vi "Qudi_HiM_QPD_PID.vi"(3 "N Z positions":i32) -> ()   [LabVIEW 2015]
uses:
  <vilib>/rvi/Analysis/control/PID/Typedef/niFpgaPID_PIGains.ctl
  <vilib>/Platform/TimedLoop/XDataNode/timing_clust.ctl
  <vilib>/Platform/TimedLoop/XDataNode/nitl_modes.ctl
  <vilib>/Platform/TimedLoop/XDataNode/wakeup.ctl
  <vilib>/rvi/FXPMathLib/basic elements/FxpIntAccumulator/subVIs/nifxpmath_IntAccumulator_SimConfig.ctl
  <vilib>/rvi/Emulation/niFpgaGetClockAttributes.vi
  <vilib>/rvi/Emulation/niFpgaSctlEmulationGetInTimedLoop.vi
  <vilib>/rvi/Emulation/niFpgaEmulationReportErrorSimple.vi
  <vilib>/rvi/eio/common/nirviEmuTemplateMethod_errors.vi
  <vilib>/rvi/Emulation/niFpgaProcessEmulError.vi
  <vilib>/rvi/Analysis/common/codeGenErrors/XNode/niFpgaXNodeCodeGenErrorHandle.vi
  <vilib>/rvi/Emulation/niFpgaCriticalErrorInLSC.vi
  <vilib>/rvi/FXPMathLib/basic elements/FxpIntAccumulator/simVIs/DllFxpIntAccumulator_sub.vi
  <vilib>/rvi/Analysis/control/PID/SubVIs/niFpgaPID_PIWrapper.vi
  <vilib>/eio/EIONode/EIONode.xnode
  <vilib>/rvi/Analysis/measure/dc-rms/XNode/niFpgaDC-RMS.xnode
  <vilib>/Platform/TimedLoop/XDataNode/XDataNode.xnode
  <vilib>/rvi/FXPMathLib/basic elements/FxpIntAccumulator/XNode/nifxpmath_IntAccumulator.xnode
  <vilib>/Platform/TimedLoop/XDataNode/XDNodeRunTimeDep.lvlib
panel:
  in  "exposure_time_ms":u16
  in  "integration_time_us":u32=100 caption="Count(uSec)"
  in  "stop":bool
  out "duration_ms":u32
  out "X":i16
  out "Y":i16
  out "Sum":i16
  out "counter":u32
  out "output":i16
  in  "reset":bool
  in  "reset_counter":bool
  in  "autofocus":bool
  in  "setpoint":i16
  in  "P":i16
  in  "I":i16
  in  "ref_axis":bool
  out "n cycles":i32
  out "Images acquired":i32
  in  "Laser lines":i32[](array[numeric])=[0, 0, 0, 0, 0]
  in  "Laser power":i16[](array[numeric])=[0, 0, 0, 0, 0]
  in  "N laser lines":i32
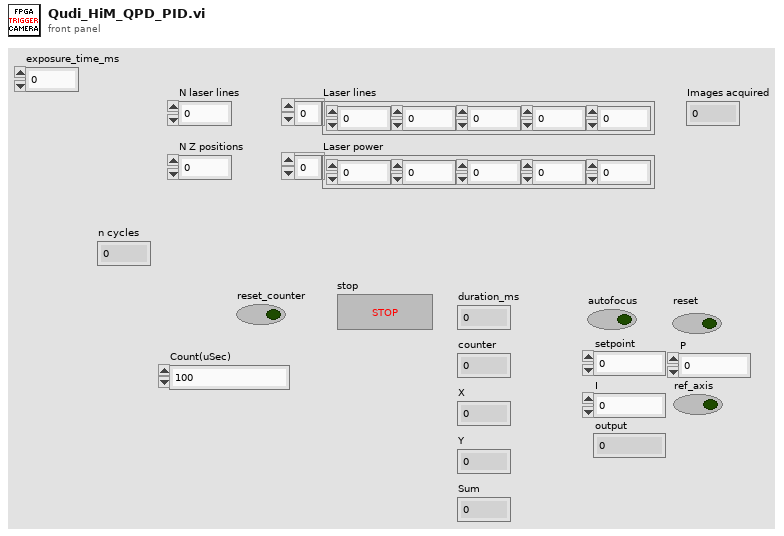
[diagram p1: front panel]
types:
  T1 = typedef "niFpgaPID_PIGains.ctl" = cluster{"proportional gain":sgl, "integral gain":sgl}
  T2 = typedef "XDNodeRunTimeDep.lvlib/timing_clust.ctl" = cluster{"Expected End [f-1]":u64, "Actual End [f-1]":u64, "Finished Late? [f-1]":bool, "Expected End [i-1]":u64, "Actual End [i-1]":u64, "Finished Late? [i-1]":bool, "Expected Start [i]":u64, "Actual Start [i]":u64, "Expected Start [f]":u64, "Actual Start [f]":u64, "Source Name":string, "Structure Name":string, "Period":i64, "Deadline":i64, "Offset":i64, "Start":i64, "Priority":i32, "Timeout":i32, "Mode":T3, "Wakeup Reason":T4, "Error":errorcluster, "Source Type":string, "Secondary Source Type":string, "Global End Time":u64, "Global Start Time":u64, "Frame Duration":u64, "Iteration Duration":u64, "Assigned CPU":i32, "I/O Scan Engine Mode":u32}
  T3 = typedef "XDNodeRunTimeDep.lvlib/nitl_modes.ctl" = enum32{"No Change", "Process missed periods, maintain original phase", "Discard missed periods, maintain original phase", "Process missed periods, ignore original phase", "Discard missed periods, ignore original phase"}
  T4 = typedef "XDNodeRunTimeDep.lvlib/wakeup.ctl" = enum32{"Normal", "Aborted", "Asynchronous wakeup", "Timing source error", "Timed loop error", "Timeout"}
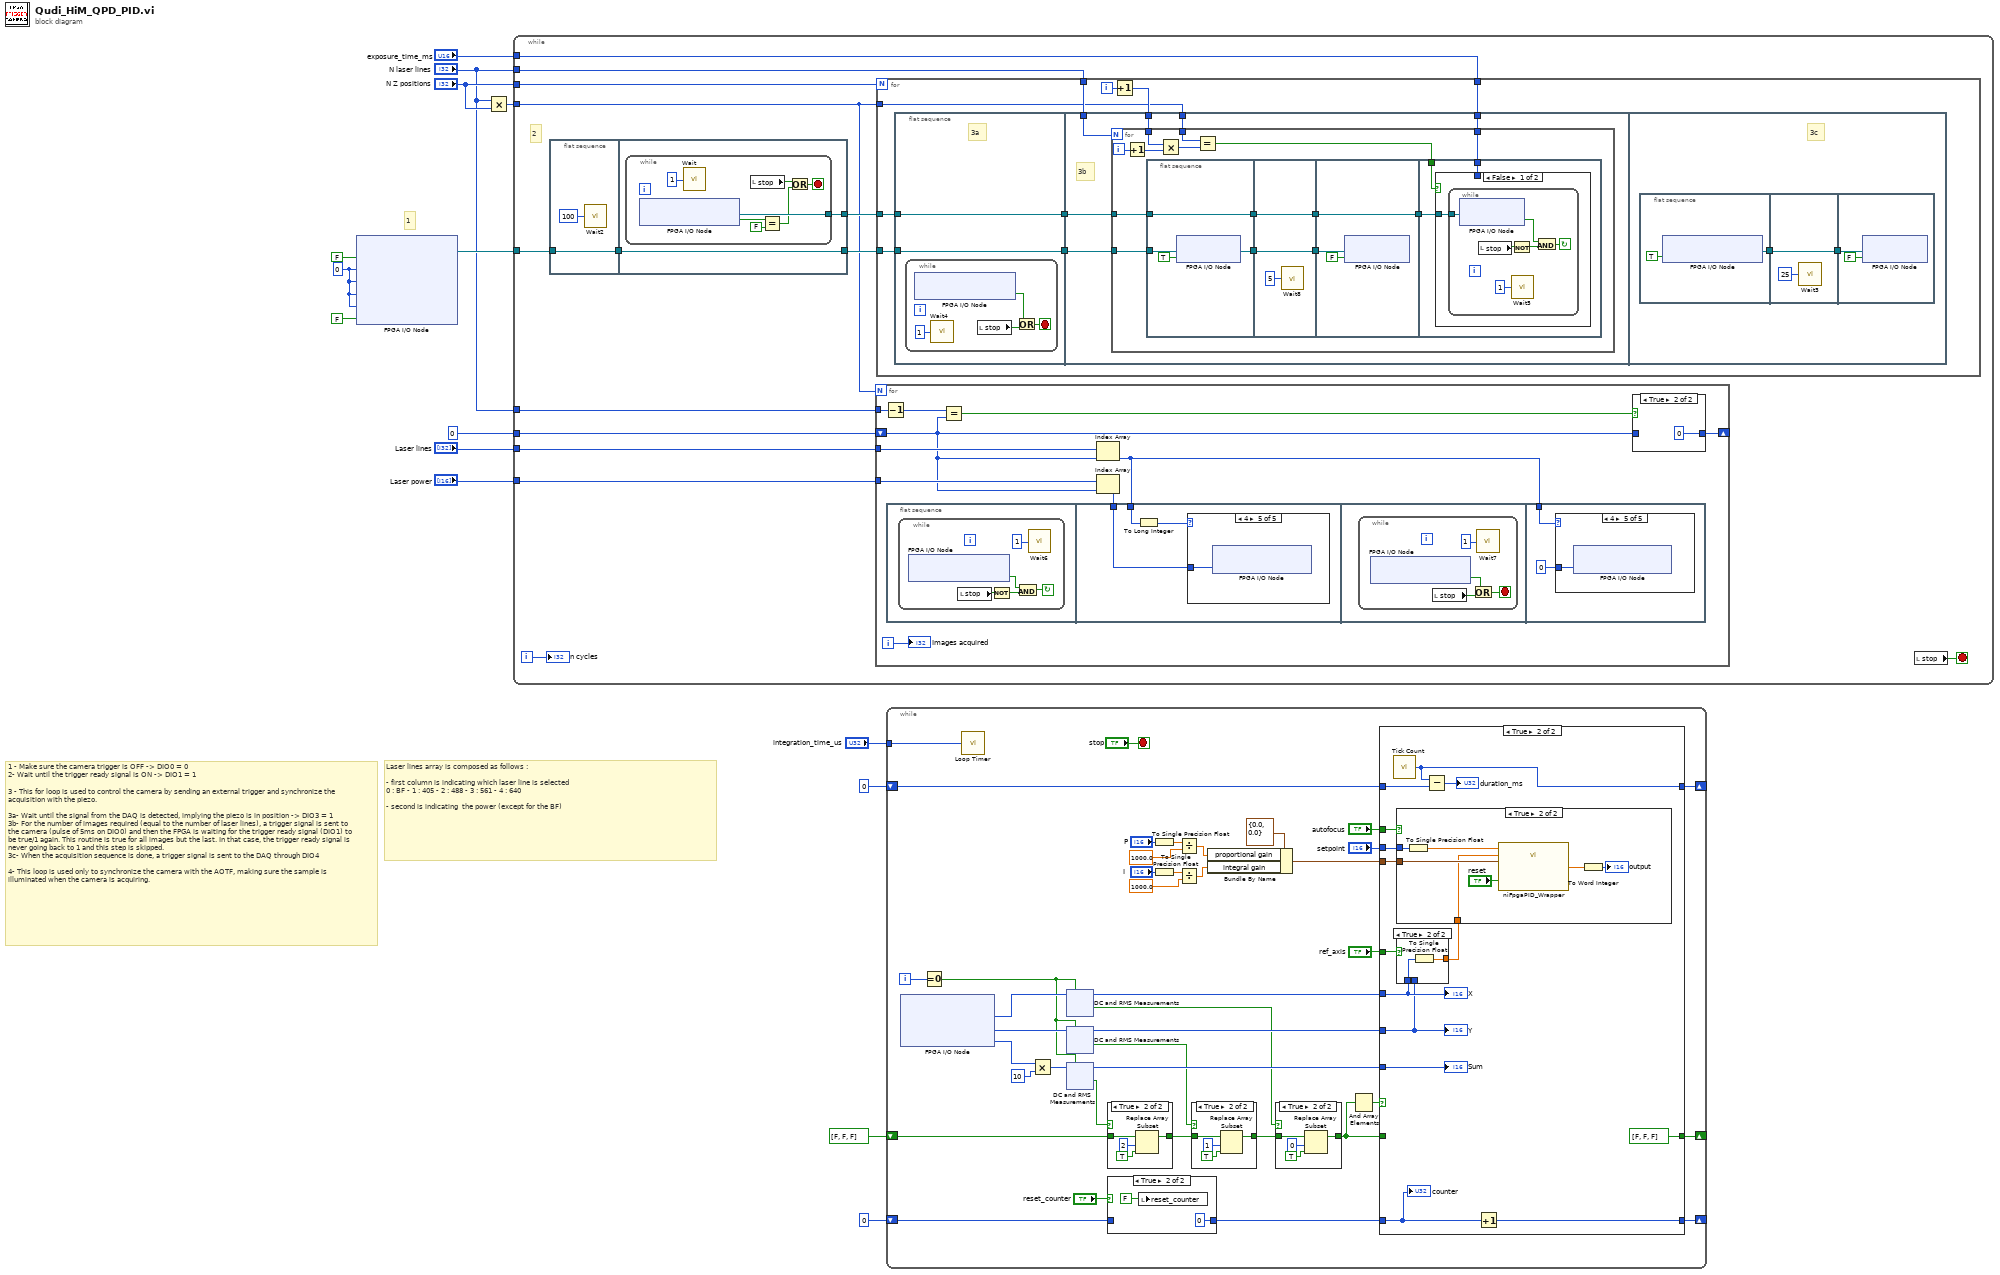
[diagram p0: block diagram]
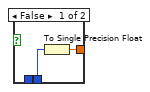
[diagram p7: hidden frame]
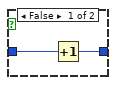
[diagram p9: hidden frame]
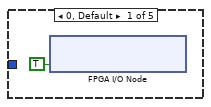
[diagram p10: hidden frame]
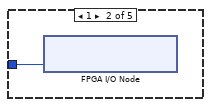
[diagram p11: hidden frame]
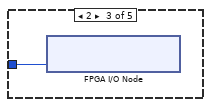
[diagram p12: hidden frame]
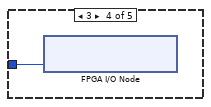
[diagram p13: hidden frame]
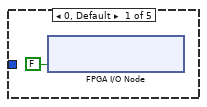
[diagram p14: hidden frame]
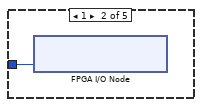
[diagram p15: hidden frame]
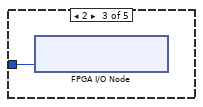
[diagram p16: hidden frame]
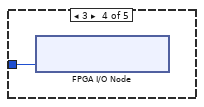
[diagram p17: hidden frame]
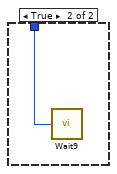
[diagram p18: hidden frame]
diagram:
  w10 = i16 0 ("Connector0/AO0")
  # "Laser lines array is composed as follows :\n\n- first column is indicating which laser line is selected \n0 : BF - 1 : 405 - 2 : 488 - 3 : 561 - 4 : 640\n\n- second is indicating  the power (except for the BF)"
  # "1"
  # "1 - Make sure the camera trigger is OFF -> DIO0 = 0\n2- Wait until the trigger ready signal is ON -> DIO1 = 1\n\n3 - This for loop is used to control the camera by sending an external trigger and synchronize the acquisition with the piezo.\n\n3a- Wait until the signal from the DAQ is detected, implying the piezo is in position -> DIO3 = 1 \n3b- For the number of images required (equal to the number of laser lines), a trigger signal is sent to the camera (pulse of 5ms on DIO0) and then the FPGA is waiting for the trigger ready signal (DIO1) to be true/1 again. This routine is true for all images but the last. In that case, the trigger ready signal is never going back to 1 and this step is skipped. \n3c- When the acquisition sequence is done, a trigger signal is sent to the DAQ through DIO4\n\n4- This loop is used only to synchronize the camera with the AOTF, making sure the sample is illuminated when the camera is acquiring."
  n1 = xnode "FPGA I/O Node"("Connector0/DIO0"=FALSE, "Connector0/AO0"=w10, "Connector0/AO1"=w10, "Connector0/AO2"=w10, "Connector0/AO3"=w10, "Connector0/DIO5"=FALSE) -> ("FPGA I/O Out"=w14:refnum<k21>)  [unwired: 6 in, 5 out]
  n2 = Multiply(x="N laser lines", y="N Z positions") -> (x*y=w3:i32)
  n3 = while {
    tunnel: w14 -> [w28]
    tunnel: "Laser power" -> [w25]
    tunnel: "Laser lines" -> [w24]
    tunnel: 0 -> [w23]
    tunnel: "N Z positions" -> [w22]
    tunnel: "N laser lines" -> [w19]
    tunnel: w3 -> [w18]
    tunnel: "N laser lines" -> [w17]
    tunnel: "exposure_time_ms" -> [w16]
    i -> [w20]
    stop <- w21 stop-if-true
    # "2"
    n4 = flat-sequence {
      tunnel: w28 -> [w68]
      tunnel: [w68] -> w29
      tunnel: w29 -> [w70]
      tunnel: [w70] -> w27
      tunnel: [w69] -> w26
      frame #0 {
        n5 = call "Wait2"("Count(uSec)"=u8 100 ("Count(mSec)")) -> ()  [unwired: 1 out]
      }
      frame #1 {
        n6 = while {
          tunnel: [w77] -> w69
          stop <- w72 stop-if-true
          n7 = xnode "FPGA I/O Node"() -> ("Connector0/DIO1"=w76:bool, "FPGA I/O Out"=w77:refnum<k21>)  [unwired: 1 in]
          n8 = call "Wait"("Count(mSec)"=u8 1) -> ()  [unwired: 1 out]
          n9 = local read "stop"() -> (w73:bool)
          n10 = Equal?(x=w76, y=FALSE) -> (x = y?=w74:bool)
          n11 = Or(x=w73, y=w74) -> (x .or. y?=w72:bool)
        }
      }
    }
    n12 = for {
      N: w18 -> [_]
      shift-right: [w37] -> _
      shift-left: w23 -> [w34]
      tunnel: w24 -> [w36]
      tunnel: w25 -> [w35]
      tunnel: w17 -> [w32]
      i -> [w30]
      n13 = Decrement(x=w32) -> (x-1=w31:i32)
      n14 = flat-sequence {
        tunnel: w39 -> [w49]
        tunnel: w33 -> [w48]
        tunnel: w39 -> [w60]
        frame #0 {
          n15 = while {
            stop <- w44 continue-if-true
            n16 = xnode "FPGA I/O Node"() -> ("Connector0/DIO2"=w45:bool)  [unwired: 1 in, 1 out]
            n17 = local read "stop"() -> (w46:bool)
            n18 = Not(x=w46) -> (.not. x?=w47:bool)
            n19 = And(x=w45, y=w47) -> (x .and. y?=w44:bool)
            n20 = call "Wait6"("Count(mSec)"=u8 1) -> ()  [unwired: 1 out]
          }
        }
        frame #1 {
          n21 = To Long Integer(number=w49) -> (32bit integer=w50:i32)
          n22 = case shown="4" w50 {
            tunnel: w48 -> [_ w52 w53 w54 w55]
            frame 0, Default {
              n23 = xnode "FPGA I/O Node"("Connector0/DIO5"=TRUE) -> ()  [unwired: 1 in, 1 out]
            }
            frame 1 {
              n24 = xnode "FPGA I/O Node"("Connector0/AO2"=w52) -> ()  [unwired: 1 in, 1 out]
            }
            frame 2 {
              n25 = xnode "FPGA I/O Node"("Connector0/AO3"=w53) -> ()  [unwired: 1 in, 1 out]
            }
            frame 3 {
              n26 = xnode "FPGA I/O Node"("Connector0/AO0"=w54) -> ()  [unwired: 1 in, 1 out]
            }
            frame 4 {
              n27 = xnode "FPGA I/O Node"("Connector0/AO1"=w55) -> ()  [unwired: 1 in, 1 out]
            }
          }
        }
        frame #2 {
          n28 = while {
            stop <- w57 stop-if-true
            n29 = xnode "FPGA I/O Node"() -> ("Connector0/DIO2"=w58:bool)  [unwired: 1 in, 1 out]
            n30 = local read "stop"() -> (w59:bool)
            n31 = Or(x=w58, y=w59) -> (x .or. y?=w57:bool)
            n32 = call "Wait7"("Count(mSec)"=u8 1) -> ()  [unwired: 1 out]
          }
        }
        frame #3 {
          n33 = case shown="4" w60 {
            tunnel: i16 0 -> [_ w63 w64 w65 w66]
            frame 0, Default {
              n34 = xnode "FPGA I/O Node"("Connector0/DIO5"=FALSE) -> ()  [unwired: 1 in, 1 out]
            }
            frame 1 {
              n35 = xnode "FPGA I/O Node"("Connector0/AO2"=w63) -> ()  [unwired: 1 in, 1 out]
            }
            frame 2 {
              n36 = xnode "FPGA I/O Node"("Connector0/AO3"=w64) -> ()  [unwired: 1 in, 1 out]
            }
            frame 3 {
              n37 = xnode "FPGA I/O Node"("Connector0/AO0"=w65) -> ()  [unwired: 1 in, 1 out]
            }
            frame 4 {
              n38 = xnode "FPGA I/O Node"("Connector0/AO1"=w66) -> ()  [unwired: 1 in, 1 out]
            }
          }
        }
      }
      n39 = Equal?(x=w31, y=w34) -> (x = y?=w38:bool)
      n40 = Index Array(array=w36, index=w34) -> (element=w39:i32)
      n41 = Index Array(array=w35, index=w34) -> (element=w33:i16)
      n42 = case shown="True" w38 {
        tunnel: w34 -> [w41 _]
        tunnel: [w40 0] -> w37
        frame False {
          n43 = Increment(x=w41) -> (x+1=w40:i32)
        }
        frame True {
        }
      }
      "Images acquired" <- w30
    }
    n44 = for {
      N: w22 -> [_]
      tunnel: w27 -> [w85]
      tunnel: w26 -> [w86]
      tunnel: w19 -> [w81]
      tunnel: w18 -> [w79]
      tunnel: w16 -> [w78]
      i -> [w82]
      n45 = flat-sequence {
        tunnel: w85 -> [w87]
        tunnel: w86 -> [w88]
        tunnel: [w88] -> w84
        tunnel: [w87] -> w83
        tunnel: w84 -> [w98]
        tunnel: w83 -> [w97]
        tunnel: w81 -> [w96]
        tunnel: w80 -> [w95]
        tunnel: w79 -> [w94]
        tunnel: w78 -> [w93]
        frame #0 {
          # "3a"
          n46 = while {
            stop <- w90 stop-if-true
            n47 = xnode "FPGA I/O Node"() -> ("Connector0/DIO3"=w91:bool)  [unwired: 1 in, 1 out]
            n48 = call "Wait4"("Count(mSec)"=u8 1) -> ()  [unwired: 1 out]
            n49 = local read "stop"() -> (w92:bool)
            n50 = Or(x=w91, y=w92) -> (x .or. y?=w90:bool)
          }
        }
        frame #1 {
          # "3b"
          n51 = for {
            N: w96 -> [_]
            tunnel: w98 -> [w107]
            tunnel: w97 -> [w106]
            tunnel: w95 -> [w103]
            tunnel: w94 -> [w101]
            tunnel: w93 -> [w99]
            i -> [w105]
            n52 = Increment(x=w105) -> (x+1=w104:i32)
            n53 = flat-sequence {
              tunnel: [w115] -> w112
              tunnel: [w113] -> w111
              tunnel: w106 -> [w114]
              tunnel: w107 -> [w113]
              tunnel: w112 -> [w119]
              tunnel: [w119] -> w110
              tunnel: [w118] -> w109
              tunnel: w111 -> [w118]
              tunnel: w110 -> [w121]
              tunnel: [w120] -> w108
              tunnel: w109 -> [w120]
              tunnel: w108 -> [w125]
              tunnel: w100 -> [w124]
              tunnel: w99 -> [w123]
              frame #0 {
                n54 = xnode "FPGA I/O Node"("I/O Item"=TRUE ("Connector0/DIO0"), "FPGA I/O In"=w114) -> ("FPGA I/O Out"=w115:refnum<k21>)
              }
              frame #1 {
                n55 = call "Wait8"("Count(mSec)"=u8 5) -> ()  [unwired: 1 out]
              }
              frame #2 {
                n56 = xnode "FPGA I/O Node"("I/O Item"=FALSE ("Connector0/DIO0"), "FPGA I/O In"=w121) -> ()  [unwired: 1 out]
              }
              frame #3 {
                n57 = case shown="False" w124 {
                  tunnel: w125 -> [w126 _]
                  tunnel: w123 -> [_ w133]
                  frame False {
                    n58 = while {
                      tunnel: w126 -> [w132]
                      stop <- w128 continue-if-true
                      n59 = xnode "FPGA I/O Node"("FPGA I/O In"=w132) -> ("I/O Item"=w129:bool)  [unwired: 1 out]
                      n60 = local read "stop"() -> (w131:bool)
                      n61 = Not(x=w131) -> (.not. x?=w130:bool)
                      n62 = call "Wait5"("Count(mSec)"=u8 1) -> ()  [unwired: 1 out]
                      n63 = And(x=w129, y=w130) -> (x .and. y?=w128:bool)
                    }
                  }
                  frame True {
                    n64 = call "Wait9"("Count(mSec)"=w133) -> ()  [unwired: 1 out]
                  }
                }
              }
            }
            n65 = Multiply(x=w103, y=w104) -> (x*y=w102:i32)
            n66 = Equal?(x=w101, y=w102) -> (x = y?=w100:bool)
          }
        }
        frame #2 {
          # "3c"
          n67 = flat-sequence {
            tunnel: [w137] -> w135
            tunnel: w135 -> [w138]
            tunnel: [w138] -> w134
            tunnel: w134 -> [w140]
            frame #0 {
              n68 = xnode "FPGA I/O Node"("Connector0/DIO4"=TRUE) -> ("FPGA I/O Out"=w137:refnum<k21>)  [unwired: 1 in]
            }
            frame #1 {
              n69 = call "Wait3"("Count(mSec)"=u8 25) -> ()  [unwired: 1 out]
            }
            frame #2 {
              n70 = xnode "FPGA I/O Node"("I/O Item"=FALSE ("Connector0/DIO0"), "FPGA I/O In"=w140) -> ()  [unwired: 1 out]
            }
          }
        }
      }
      n71 = Increment(x=w82) -> (x+1=w80:i32)
    }
    n72 = local read "stop"() -> (w21:bool)
    "n cycles" <- w20
  }
  n73 = while {
    shift-right: [w165] -> _
    shift-left: bool[] [FALSE, FALSE, FALSE] ("initialized array") -> [w173]
    shift-right: [w163] -> _
    shift-left: u32 0 -> [w164]
    tunnel: "integration_time_us" -> [w162]
    shift-right: [w161] -> _
    shift-left: u32 0 -> [w159]
    i -> [w179]
    stop <- "stop" stop-if-true
    n74 = xnode "FPGA I/O Node"() -> ("Connector0/AI0"=w181:i16, "Connector0/AI1"=w177:i16, "Connector0/AI2"=w144:i16)  [unwired: 3 in, 3 out]
    n75 = Equal To 0?(x=w179) -> (x = 0?=w174:bool)
    n76 = call "Loop Timer"("Count(uSec)"=w162) -> ()  [unwired: 1 out]
    n77 = Multiply(x=w144, y=i16 10) -> (x*y=w143:i16)
    n78 = xnode "DC and RMS Measurements"("input data"=w181, "reset"=w174) -> ("DC"=w178:i16, "output valid"=w168:bool)
    n79 = xnode "DC and RMS Measurements"("input data"=w177, "reset"=w174) -> ("DC"=w176:i16, "output valid"=w169:bool)
    n80 = xnode "DC and RMS Measurements"("input data"=w143, "reset"=w174) -> ("DC"=w175:i16, "output valid"=w170:bool)
    n81 = case shown="True" w170 {
      tunnel: w173 -> [w190 w193]
      tunnel: [w190 w191] -> w172
      frame False {
      }
      frame True {
        n82 = Replace Array Subset(array=w193, new element=TRUE, index=2) -> (w191:bool[])
      }
    }
    n83 = case shown="True" "reset_counter" {
      tunnel: w159 -> [w182 _]
      tunnel: [w182 u32 0] -> w158
      frame False {
      }
      frame True {
        n84 = local write "reset_counter"(FALSE ("Reset counter")) -> ()
      }
    }
    n85 = To Single Precision Float(number="P") -> (single precision float=w151:sgl)
    n86 = To Single Precision Float(number="I") -> (single precision float=w148:sgl)
    n87 = Divide(x=w151, y=sgl 1000.0) -> (x/y=w149:sgl)
    n88 = Divide(x=w148, y=sgl 1000.0) -> (x/y=w146:sgl)
    n89 = case shown="True" w169 {
      tunnel: w172 -> [w195 w198]
      tunnel: [w195 w196] -> w171
      frame False {
      }
      frame True {
        n90 = Replace Array Subset(array=w198, new element=TRUE, index=1) -> (w196:bool[])
      }
    }
    n91 = Bundle By Name(cluster=T1 {"proportional gain"=0.0, "integral gain"=0.0} ("gains"), "proportional gain"=w149, "integral gain"=w146) -> (w152:T1)
    n92 = case shown="True" w168 {
      tunnel: [w185 w187] -> w166
      tunnel: w171 -> [w185 w186]
      frame False {
      }
      frame True {
        n93 = Replace Array Subset(array=w186, new element=TRUE, index=0) -> (w187:bool[])
      }
    }
    n94 = And Array Elements(Boolean array=w166) -> (logical AND=w167:bool)
    n95 = case shown="True" w167 {
      tunnel: w178 -> [_ w205]
      tunnel: w176 -> [_ w203]
      tunnel: w175 -> [_ w211]
      tunnel: w166 -> [w202 _]
      tunnel: [w202 bool[] [FALSE, FALSE, FALSE] ("initialized array")] -> w165
      tunnel: w164 -> [w201 w215]
      tunnel: [w201 w213] -> w163
      tunnel: w158 -> [w200 w210]
      tunnel: [w200 w212] -> w161
      tunnel: "autofocus" -> [_ w209]
      tunnel: "setpoint" -> [_ w208]
      tunnel: w152 -> [_ w207]
      tunnel: "ref_axis" -> [_ w206]
      frame False {
      }
      frame True {
        n96 = call "Tick Count"() -> ("Tick Count(mSec)"=w213:u32)
        n97 = case shown="True" w206 {
          tunnel: w205 -> [_ w220]
          tunnel: [w217 w219] -> w204
          tunnel: w203 -> [w218 _]
          frame False {
            n98 = To Single Precision Float(number=w218) -> (single precision float=w217:sgl)
          }
          frame True {
            n99 = To Single Precision Float(number=w220) -> (single precision float=w219:sgl)
          }
        }
        n100 = case shown="True" w209 {
          tunnel: w208 -> [_ w227]
          tunnel: w207 -> [_ w225]
          tunnel: w204 -> [_ w221]
          frame False {
          }
          frame True {
            n101 = To Single Precision Float(number=w227) -> (single precision float=w226:sgl)
            n102 = call-poly <vilib>:"niFpgaPID_Wrapper.vi"("setpoint"=w226, "reset? (F)"="reset", "process variable"=w221, "gains"=w225) -> ("output"=w223:sgl)  [unwired: 9 in, 2 out]
            n103 = To Word Integer(number=w223) -> (16bit integer=→"output":i16)
          }
        }
        n104 = Subtract(x=w213, y=w215) -> (x-y=→"duration_ms":u32)
        n105 = Increment(x=w210) -> (x+1=w212:u32)
        "X" <- w205
        "Y" <- w203
        "Sum" <- w211
        "counter" <- w210
      }
    }
  }
